vi "get justification.vi"(8 "error in (no error)":errorcluster, 11 "String Control in":refnum<class "String Control.lvclass">) -> (0 "error out":errorcluster, 2 "String Text.Justification":enum16{"Left", "Center", "Right"}(ring), 3 "String Control out":refnum<class "String Control.lvclass">)   [LabVIEW 2010, in "String Control.lvclass"]
uses:
  String Control.lvclass
  String Control.lvclass/String Control.ctl
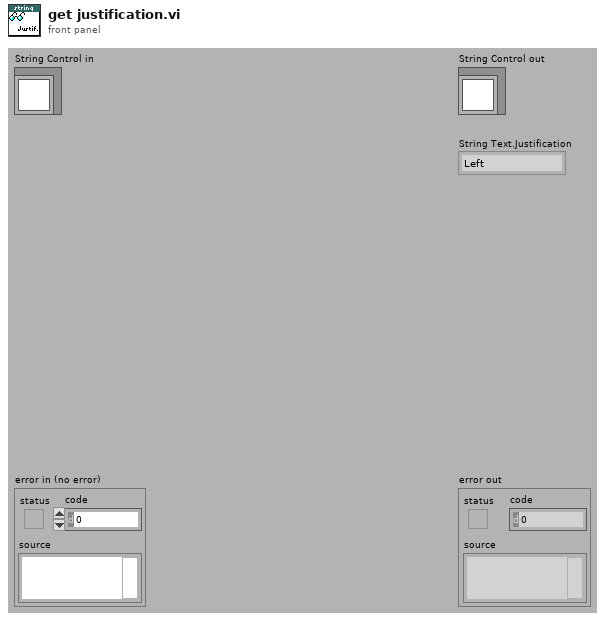
[diagram p1: front panel]
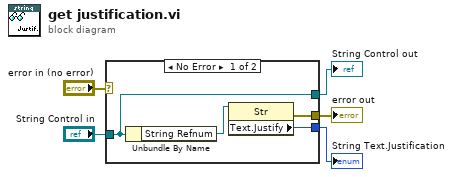
[diagram p0: block diagram]
diagram:
  n1 = case shown="No Error" "error in (no error)" {
    selector: "error in (no error)" -> [_ w11]
    tunnel: [w7 w11] -> w4
    tunnel: [w9 w10] -> w2
    tunnel: "String Control in" -> [w9 w10]
    tunnel: [w6 _] -> w1
    frame No Error {
      n2 = Unbundle By Name(w9) -> ("String Refnum"=w8:refnum<vi>)
      n3 = property class="Str"(reference=w8) -> (error out=w7:errorcluster, "Text.Justify"=w6:enum16{"Left", "Center", "Right"})  [unwired: 1 in, 1 out]
    }
    frame Error {
    }
  }
  "error out" <- w4
  "String Control out" <- w2
  "String Text.Justification" <- w1
